vi "Referenzfahrt beendet.vi"() -> (3 "Ref. beendet":bool)   [LabVIEW 2014]
uses:
  <vilib>/CANopenLib/CANOPEN.llb/CANopen SDO Create.vi
  <vilib>/CANopenLib/CANOPEN.llb/CANopen SDO Read [U32].vi
  <vilib>/CANopenLib/CANOPEN.llb/CANopen SDO Close.vi
panel:
  out "error out":errorcluster
  in  "Fehler (Eingang, kein Fehler)":errorcluster
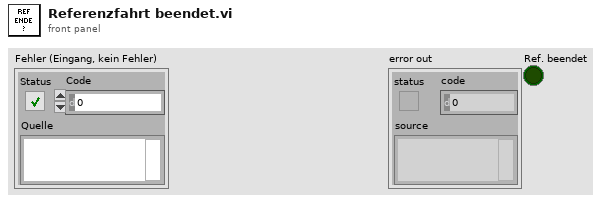
[diagram p1: front panel]
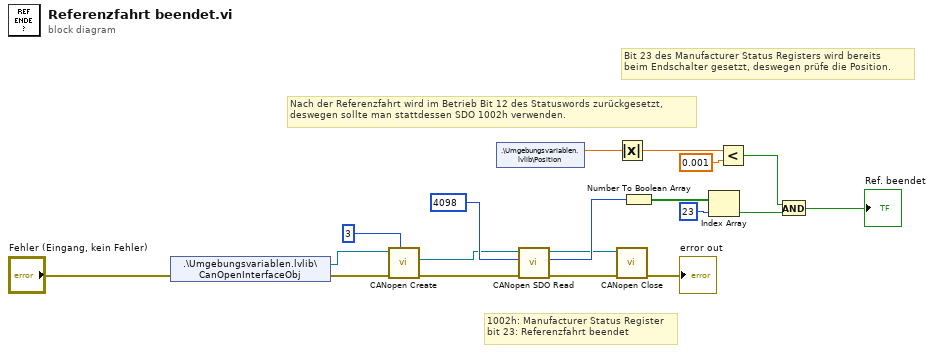
[diagram p0: block diagram]
diagram:
  # "Nach der Referenzfahrt wird im Betrieb Bit 12 des Statuswords zurückgesetzt, \ndeswegen sollte man stattdessen SDO 1002h verwenden."
  # "1002h: Manufacturer Status Register\nbit 23: Referenzfahrt beendet"
  # "Bit 23 des Manufacturer Status Registers wird bereits \nbeim Endschalter gesetzt, deswegen prüfe die Position."
  n1 = shared-variable ".\\Umgebungsvariablen.lvlib\\CanOpenInterfaceObj"(error in="Fehler (Eingang, kein Fehler)") -> (w15:refnum<k20>, error out=w16:errorcluster)
  n2 = call-poly <vilib>:"CANopen Create.vi"("node-ID"=u8 3, "error in (no error)"=w16, "interface object in"=w15) -> ("error out"=w9:errorcluster, "SDO object out"=w10:refnum<k20>)  [unwired: 6 in, 1 out]
  n3 = shared-variable ".\\Umgebungsvariablen.lvlib\\Position"() -> (w18:dbl)  [unwired: 1 in, 1 out]
  n4 = call-poly <vilib>:"CANopen SDO Read.vi"("error in (no error)"=w9, "object index"=u16 4098, "SDO object in"=w10) -> ("error out"=w7:errorcluster, "U32 data"=w13:u32, "SDO object out"=w6:refnum<k20>)  [unwired: 5 in, 1 out]
  n5 = Absolute Value(x=w18) -> (abs(x)=w17:dbl)
  n6 = call-poly <vilib>:"CANopen Close.vi"("error in (no error)"=w7, "SDO object in"=w6) -> ("error out"=→"error out":errorcluster)  [unwired: 9 in]
  n7 = Number To Boolean Array(number=w13) -> (Boolean array=w12:bool[])
  n8 = Index Array(array=w12, index=23 ("Index")) -> (element=w2:bool)
  n9 = Less?(x=w17, y=0.001) -> (x < y?=w1:bool)
  n10 = And(x=w1, y=w2) -> (x .and. y?=→"Ref. beendet":bool)
